vi "Pre Launch Init.vi"(11 "Welcome in":refnum<class "Welcome.lvclass">) -> (0 "error out":errorcluster, 3 "Welcome out":refnum<class "Welcome.lvclass">)   [LabVIEW 2015, in "Item Actor.lvlib" / "Welcome.lvclass"]
doc: "(<B>Filename</B>: Actor Framework.lvlib:Actor.lvclass:Pre Launch Init.vi)\n\nDefines behavior that occurs after the Launch Nested Actor method is invoked but before the actor's Actor Core method begins running.\n\nBy default, this method does nothing. A descendant class may override it to define behavior."
uses:
  Welcome.lvclass
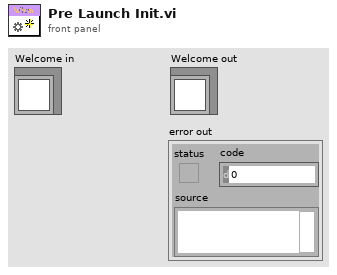
[diagram p1: front panel]
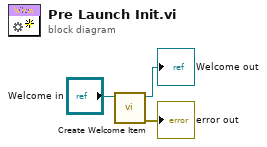
[diagram p0: block diagram]
diagram:
  n1 = call "Create Welcome Item.vi"("Welcome in"="Welcome in") -> ("error out"=→"error out":errorcluster, "Welcome out"=→"Welcome out":refnum<class "Welcome.lvclass">)  [unwired: 9 in]
